vi "Test.vi"() -> ()   [LabVIEW 2023]
uses:
  C:/Projects/Cutiss/SequenceManager/SequenceManager/LabViewWrapper/build/Easy.SequenceManager.dll
  build/Easy.SequenceManager.dll
panel:
  in  "error in (no error)":errorcluster
  out "error out":errorcluster
  out "GetNextStepsToExecuteAsJson 3":string
  out "GetNextStepsToExecuteAsJson 2":string
  out "GetNextStepsToExecuteAsJson":string
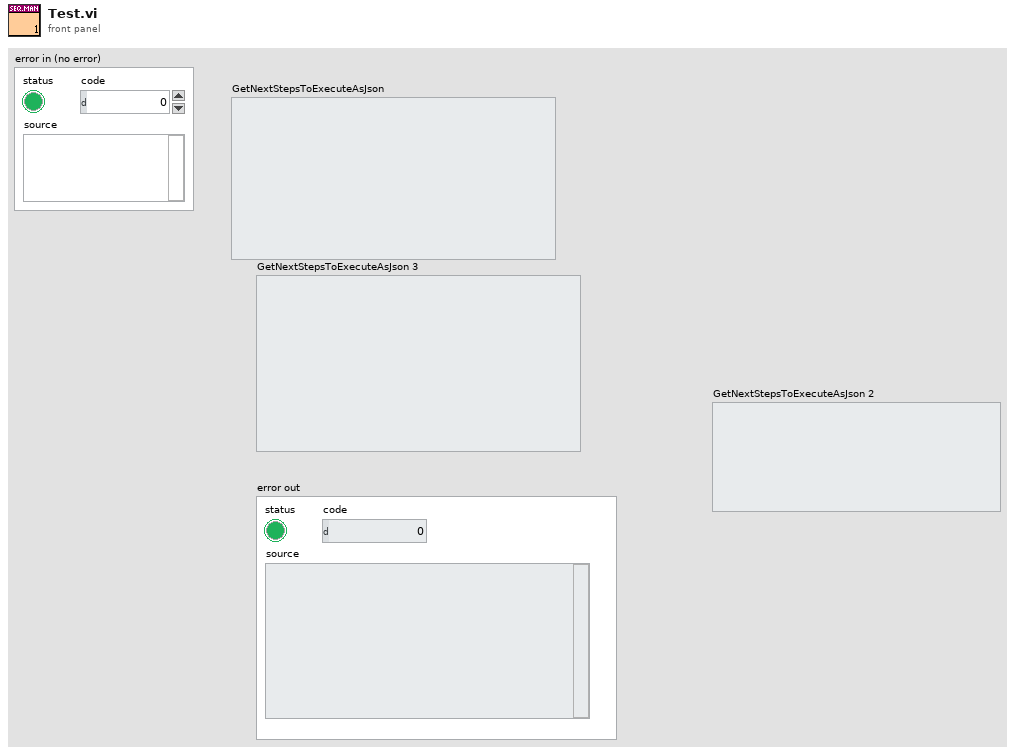
[diagram p1: front panel]
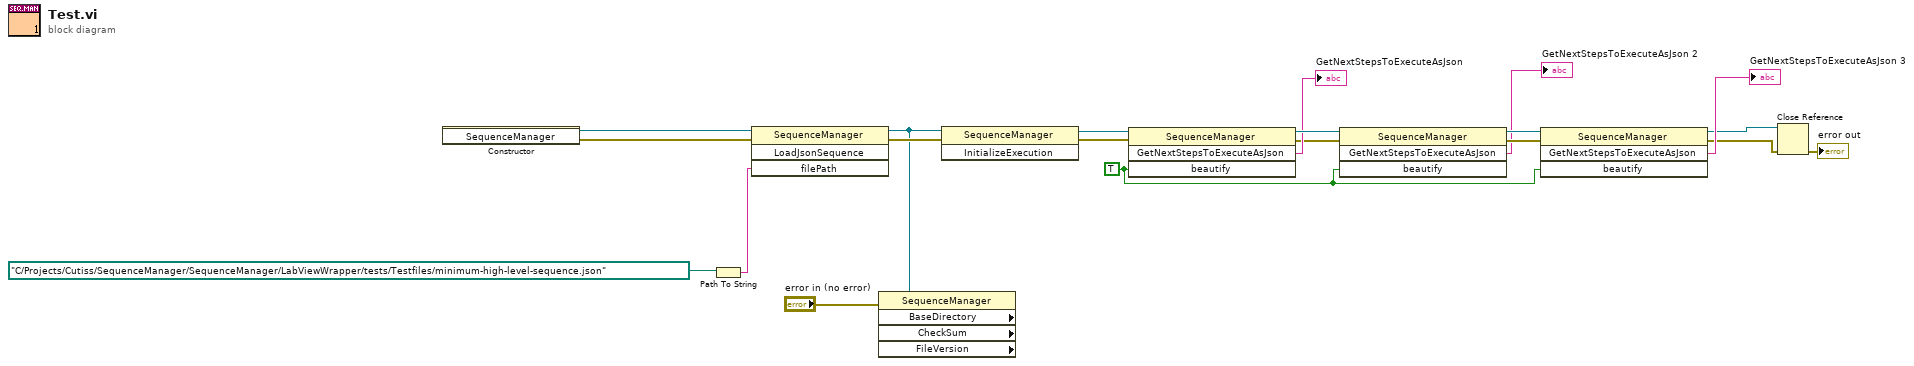
[diagram p0: block diagram]
diagram:
  w11 = TRUE ("beautify")
  n1 = constructor class="SequenceManager"() -> (reference out=w20:refnum<k24>, error out=w19:errorcluster)  [unwired: 3 in, 1 out]
  n2 = Path To String(path=path "C:/Projects/Cutiss/SequenceManager/SequenceManager/LabViewWrapper/tests/Testfiles/minimum-high-level-sequence.json") -> (string=w17:string)
  n3 = invoke class="SequenceManager" method="LoadJsonSequence"(reference=w20, error in=w19, "filePath"=w17) -> (reference out=w2:refnum<k24>, error out=w16:errorcluster)  [unwired: 1 in, 2 out]
  n4 = property class="SequenceManager" props=["BaseDirectory", "CheckSum", "FileVersion"](reference=w2, error in="error in (no error)") -> ()  [unwired: 5 out]
  n5 = invoke class="SequenceManager" method="InitializeExecution"(reference=w2, error in=w16) -> (reference out=w15:refnum<k24>, error out=w4:errorcluster)  [unwired: 1 in, 1 out]
  n6 = invoke class="SequenceManager" method="GetNextStepsToExecuteAsJson"(reference=w15, error in=w4, "beautify"=w11) -> (reference out=w14:refnum<k24>, error out=w3:errorcluster, "GetNextStepsToExecuteAsJson"=→"GetNextStepsToExecuteAsJson":string)  [unwired: 1 in, 1 out]
  n7 = invoke class="SequenceManager" method="GetNextStepsToExecuteAsJson"(reference=w14, error in=w3, "beautify"=w11) -> (reference out=w13:refnum<k24>, error out=w12:errorcluster, "GetNextStepsToExecuteAsJson"=→"GetNextStepsToExecuteAsJson 2":string)  [unwired: 1 in, 1 out]
  n8 = invoke class="SequenceManager" method="GetNextStepsToExecuteAsJson"(reference=w13, error in=w12, "beautify"=w11) -> (reference out=w6:refnum<k24>, error out=w7:errorcluster, "GetNextStepsToExecuteAsJson"=→"GetNextStepsToExecuteAsJson 3":string)  [unwired: 1 in, 1 out]
  n9 = Close Reference(reference=w6, error in (no error)=w7) -> (error out=→"error out":errorcluster)
